vi "Stop Rx With Report.vi"(8 "error in (no error)":errorcluster) -> (0 "error out":errorcluster, 3 "return type":i32)   [LabVIEW 2014, in "QCA_DUT_Func.lvlib"]
doc: "DLL_QMSL_AEROFLEX void _stdcall StopRxWithReport(int *totalPkt,int *goodPackets,int *crcErrPkt,int *rssi );"
uses:
  QCA_DUT_Func.lvlib
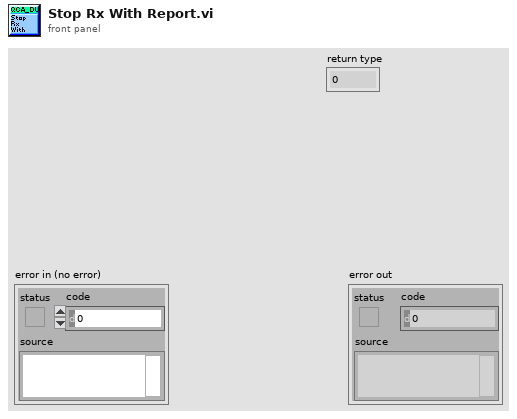
[diagram p1: front panel]
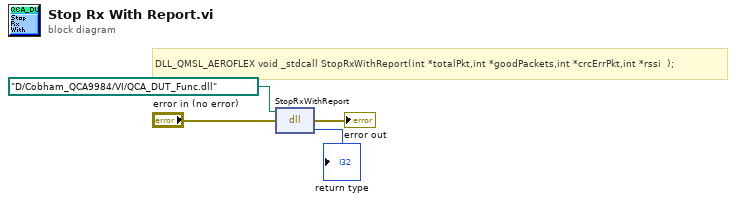
[diagram p0: block diagram]
diagram:
  # "DLL_QMSL_AEROFLEX void _stdcall StopRxWithReport(int *totalPkt,int *goodPackets,int *crcErrPkt,int *rssi  );"
  n1 = dll-call lib="D:/Cobham_QCA9984/VI/QCA_DUT_Func.dll" fn="StopRxWithReport"(path in=path "D:/Cobham_QCA9984/VI/QCA_DUT_Func.dll", error in="error in (no error)") -> (error out=→"error out":errorcluster, "return type"=→"return type":i32)  [unwired: 1 in, 1 out]
